vi "Arc Turn.vi"(0 "Speed Setpoint (0-1)":dbl format="%#_13g", 1 "Angle Radians (0 = Right)":dbl=21.5, 2 "Max Speed (TPS)":dbl format="%#_13g", 3 "Distance":dbl=21.5, 8 "Robot Width":dbl=21.5) -> (14 "Left Speed":dbl format="%#_13g", 16 "Right Speed":dbl format="%#_13g")   [LabVIEW 2015]
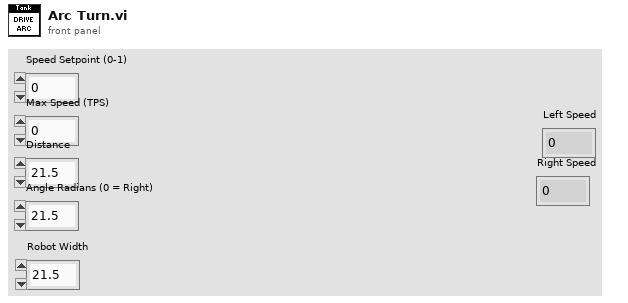
[diagram p1: front panel]
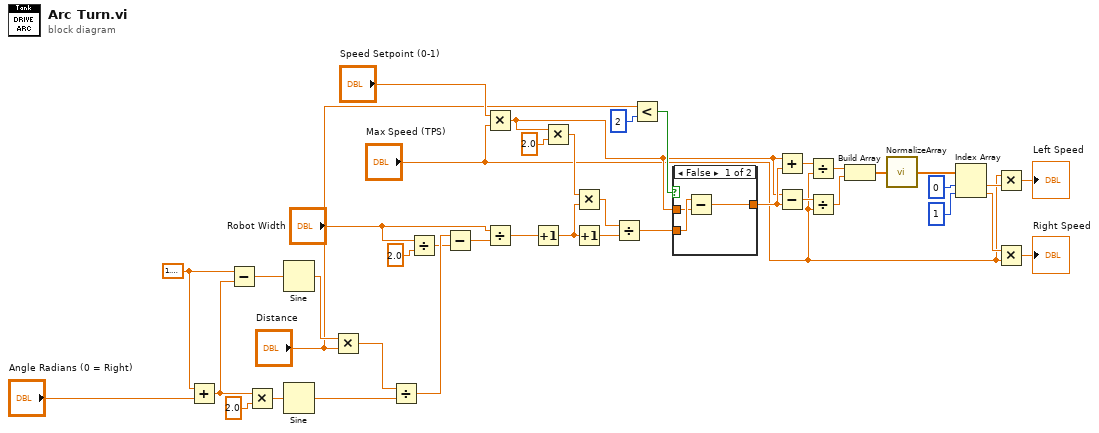
[diagram p0: block diagram]
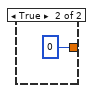
[diagram p2: hidden frame]
diagram:
  w11 = 1.5707963267948966
  n1 = Add(x=w11, y="Angle Radians (0 = Right)") -> (x+y=w12:dbl)
  n2 = Subtract(x=w11, y=w12) -> (x-y=w40:dbl)
  n3 = Multiply(x=w12, y=2.0) -> (x*y=w36:dbl)
  n4 = Sine(x=w40) -> (sin(x)=w39:dbl)
  n5 = Sine(x=w36) -> (sin(x)=w35:dbl)
  n6 = Multiply(x=w39, y="Distance") -> (x*y=w38:dbl)
  n7 = Divide(x=w38, y=w35) -> (x/y=w34:dbl)
  n8 = Divide(x="Robot Width", y=2.0) -> (x/y=w23:dbl)
  n9 = Subtract(x=w34, y=w23) -> (x-y=w33:dbl)
  n10 = Multiply(x="Speed Setpoint (0-1)", y="Max Speed (TPS)") -> (x*y=w20:dbl)
  n11 = Divide(x="Robot Width", y=w33) -> (x/y=w32:dbl)
  n12 = Increment(x=w32) -> (x+1=w27:dbl)
  n13 = Multiply(x=w20, y=2.0) -> (x*y=w29:dbl)
  n14 = Multiply(x=w29, y=w27) -> (x*y=w28:dbl)
  n15 = Increment(x=w27) -> (x+1=w26:dbl)
  n16 = Divide(x=w28, y=w26) -> (x/y=w25:dbl)
  n17 = Less?(x="Distance", y=2) -> (x < y?=w21:bool)
  n18 = case shown="False" w21 {
    tunnel: w25 -> [w43 _]
    tunnel: w20 -> [w42 _]
    tunnel: [w41 0] -> w24
    frame False {
      n19 = Subtract(x=w43, y=w42) -> (x-y=w41:dbl)
    }
    frame True {
    }
  }
  n20 = Add(x=w20, y=w24) -> (x+y=w9:dbl)
  n21 = Subtract(x=w20, y=w24) -> (x-y=w10:dbl)
  n22 = Divide(x=w9, y="Max Speed (TPS)") -> (x/y=w8:dbl)
  n23 = Divide(x=w10, y="Max Speed (TPS)") -> (x/y=w3:dbl)
  n24 = Build Array(w8, w3) -> (w2:dbl[])
  n25 = call "NormalizeArray.vi"("array"=w2) -> ("normalized array"=w1:dbl[])
  n26 = Index Array(array=w1, index #1=0 ("index"), index #2=1 ("index")) -> (element #1=w6:dbl, element #2=w13:dbl)
  n27 = Multiply(x="Max Speed (TPS)", y=w6) -> (x*y=→"Left Speed":dbl)
  n28 = Multiply(x=w13, y="Max Speed (TPS)") -> (x*y=→"Right Speed":dbl)
